vi "Condition Map Inner.vi"(6 "WiringRules[]":T1(array[ring]), 9 "Controls[]":refnum<vi>[](array[refnum]), 10 "All Terminals":i32[](array[numeric])) -> (2 "Terminal Attributes":T2)   [LabVIEW 2025, in "_Msg Rescript.lvlib" / "_Msg Rescript.lvclass"]
uses:
  _Msg Rescript.lvclass
  _Msg Rescript.lvclass/_Msg Rescript.ctl
  Attributes.ctl
  Terminal Attributes.ctl
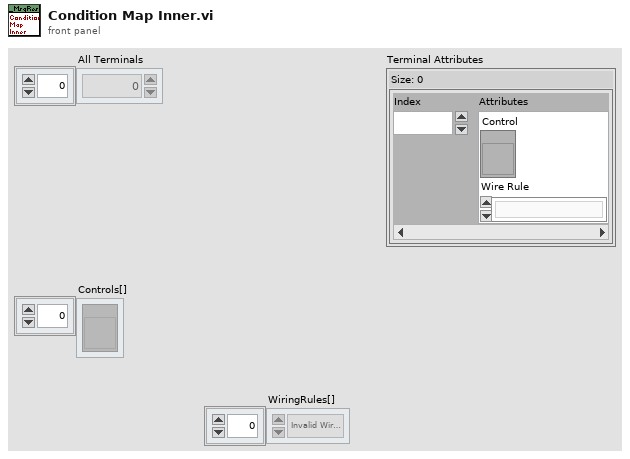
[diagram p1: front panel]
types:
  T1 = enum16{"Invalid Wire Rule", "Required", "Recommended", "Optional", "Dynamic Dispatch"}[]
  T2 = typedef "_Msg Rescript.lvlib/_Msg Rescript.lvclass/Terminal Attributes.ctl" = map{i32, T3}
  T3 = typedef "_Msg Rescript.lvlib/_Msg Rescript.lvclass/Attributes.ctl" = cluster{"Control":refnum<vi>, "Wire Rule":enum16{"Invalid Wire Rule", "Required", "Recommended", "Optional", "Dynamic Dispatch"}}
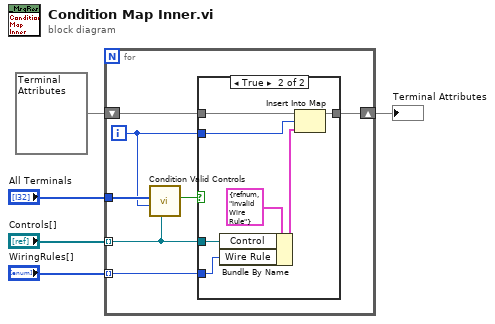
[diagram p0: block diagram]
diagram:
  n1 = for {
    tunnel: "All Terminals" -> [w8]
    shift-right: [w12] -> w3
    shift-left: T2 {} ("Msg Terminal Map") -> [w11]
    tunnel: "Controls[]" -> [w6] mode=indexing
    tunnel: "WiringRules[]" -> [w10] mode=indexing
    i -> [w7]
    n2 = call "Condition Valid Controls.vi"("Ctl Refnum"=w6, "Terminal Index"=w7, "Control Terminals"=w8) -> ("Valid"=w9:bool)  [unwired: 8 in]
    n3 = case shown="True" w9 {
      tunnel: [w13 w20] -> w12
      tunnel: w11 -> [w13 w19]
      tunnel: w10 -> [_ w18]
      tunnel: w7 -> [_ w17]
      tunnel: w6 -> [_ w16]
      frame False {
      }
      frame True {
        n4 = Bundle By Name(cluster=T3 {"Control"=refnum, "Wire Rule"=enum."Invalid Wire Rule"} ("value"), "Control"=w16, "Wire Rule"=w18) -> (w14:T3)
        n5 = Insert Into Map(map in=w19, key=w17, value=w14) -> (map out=w20:T2)  [unwired: 2 out]
      }
    }
  }
  "Terminal Attributes" <- w3
